vi "StopSubsystem.vi"(8 "error in (no error)":errorcluster, 11 "AutoDrive in":refnum<class "AutoDrive.lvclass">) -> (0 "error out":errorcluster, 3 "AutoDrive out":refnum<class "AutoDrive.lvclass">)   [LabVIEW 2017]
uses:
  AutoSubsystem/AutoSubroutine.lvclass
  AutoSubsystem/AutoDrive/AutoDrive.lvclass
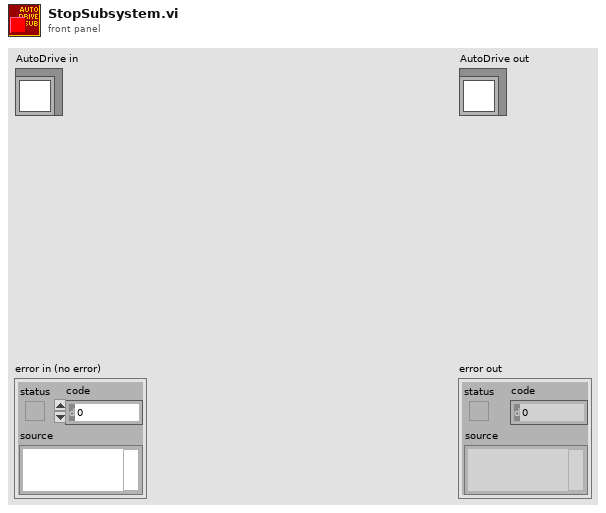
[diagram p1: front panel]
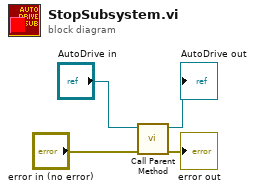
[diagram p0: block diagram]
diagram:
  n1 = call-parent "Call Parent Method"("error in (no error)"="error in (no error)", "AutoSubroutine in"="AutoDrive in") -> ("error out"=→"error out":errorcluster, "AutoSubroutine out"=→"AutoDrive out":refnum<class "AutoSubroutine.lvclass">)  [unwired: 8 in]
